vi "Enqueue Message (Single).vi"(6 "Priority Message? (F)":bool caption="우선순위 메시지? (거짓)", 8 "error in (no error)":errorcluster caption="에러 입력(에러 없음)", 9 "Message Data":variant caption="메시지 데이터", 10 "Message":string caption="메시지", 11 "Message Queue":refnum<queue> caption="메시지 큐") -> (0 "error out":errorcluster caption="에러 출력", 3 "dup Message Queue":refnum<queue> caption="메시지 큐 복제")   [LabVIEW 2018, in "Message Queue.lvlib"]
doc: "일반 메시지의 경우, 메시지를 큐에 추가합니다. 우선순위 메시지의 경우, 메시지를 큐의 앞쪽에 추가합니다."
uses:
  Message Queue.lvlib
  Message Cluster.ctl
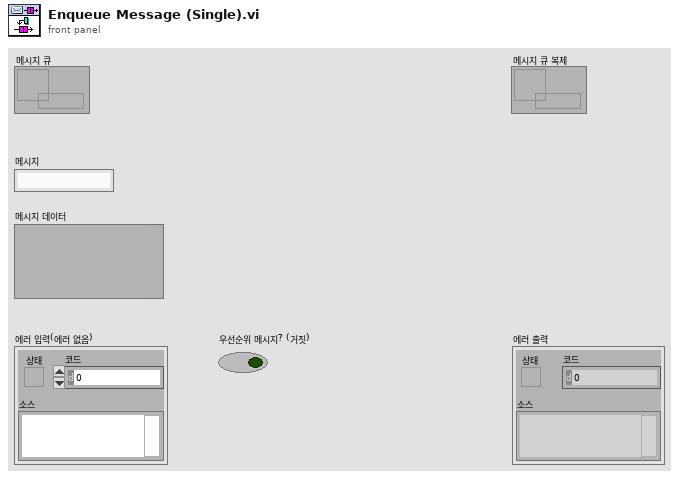
[diagram p1: front panel]
types:
  T1 = typedef "Message Queue.lvlib/Message Cluster.ctl" = cluster{"Message":string, "Message Data":variant}
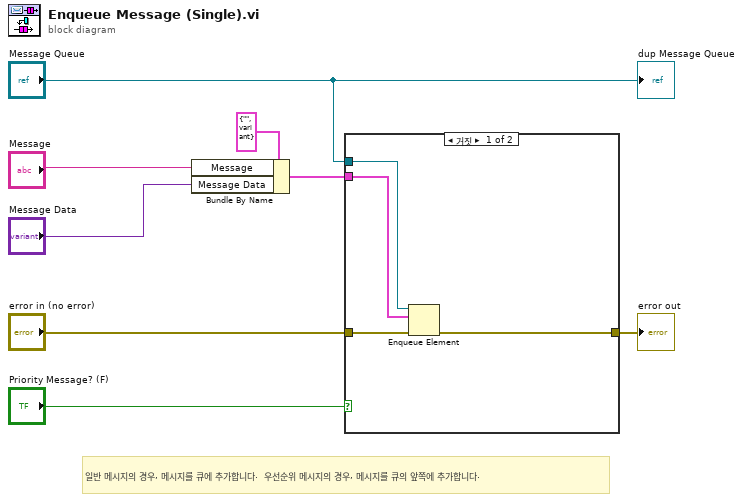
[diagram p0: block diagram]
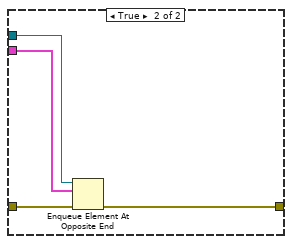
[diagram p2: hidden frame]
diagram:
  # "일반 메시지의 경우, 메시지를 큐에 추가합니다.  우선순위 메시지의 경우, 메시지를 큐의 앞쪽에 추가합니다."
  n1 = Bundle By Name(cluster=T1 {"Message"="", "Message Data"=variant} ("Message Cluster"), "Message"="Message", "Message Data"="Message Data") -> (w1:T1)
  n2 = case shown="거짓" "Priority Message? (F)" {
    tunnel: "error in (no error)" -> [w12 w16]
    tunnel: [w11 w15] -> w3
    tunnel: "Message Queue" -> [w10 w14]
    tunnel: w1 -> [w9 w13]
    frame False {
      n3 = Enqueue Element(queue=w10, element=w9, error in (no error)=w12) -> (error out=w11:errorcluster)  [unwired: 1 in, 2 out]
    }
    frame True {
      n4 = Enqueue Element At Opposite End(queue=w14, element=w13, error in (no error)=w16) -> (error out=w15:errorcluster)  [unwired: 1 in, 2 out]
    }
  }
  "error out" <- w3
  "dup Message Queue" <- "Message Queue"
